vi "Save Extra data.vi"(2 "Temps":dbl[][](array[numeric]), 3 "Pixel Num.":i32, 4 "Save data Title":T1(ring), 5 "name or relative path":path) -> ()   [LabVIEW 2024]
uses:
  <vilib>/Utility/file.llb/Write Delimited Spreadsheet (string).vi
  <vilib>/Utility/file.llb/Write Delimited Spreadsheet (DBL).vi
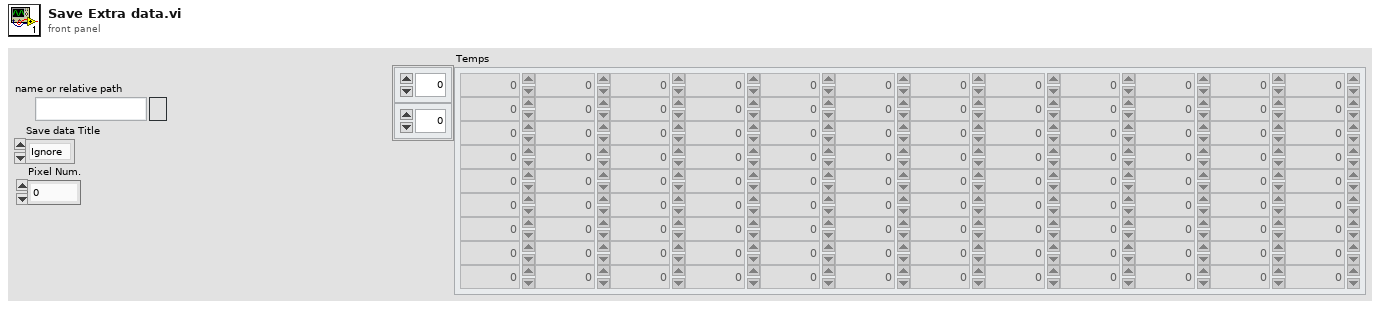
[diagram p1: front panel]
types:
  T1 = enum16{"Ignore", "All Wells Mean", "Pixel Values Wells"}
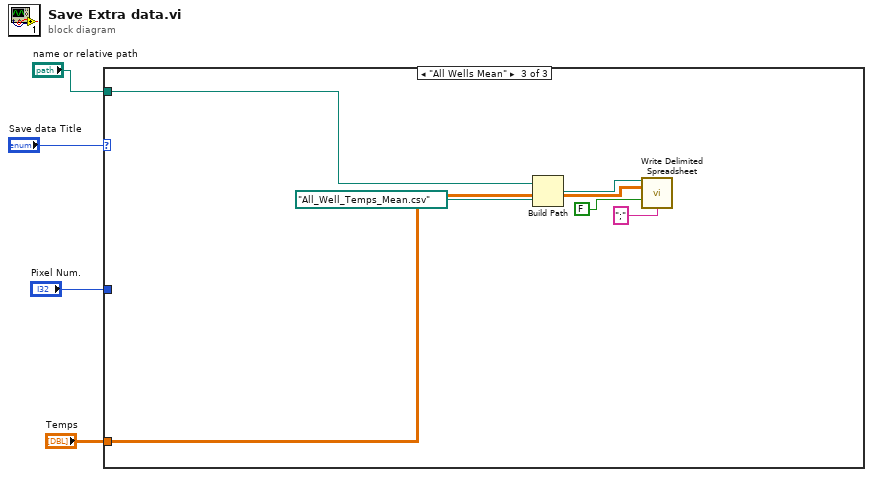
[diagram p0: block diagram]
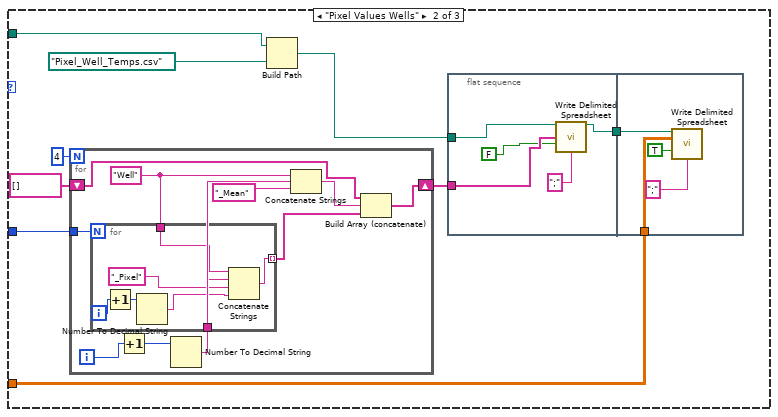
[diagram p3: hidden frame]
diagram:
  n1 = case shown="\"All Wells Mean\"" "Save data Title" {
    tunnel: "name or relative path" -> [_ w13 w43]
    tunnel: "Temps" -> [_ w9 w42]
    tunnel: "Pixel Num." -> [_ w8 _]
    frame "Ignore", Default {
    }
    frame "Pixel Values Wells" {
      n2 = for {
        N: 4 -> [_]
        tunnel: w8 -> [w23]
        shift-right: [w14] -> w6
        shift-left: string[] [] -> [w15]
        i -> [w21]
        w19 = "Well"
        n3 = Increment(x=w21) -> (x+1=w22:i32)
        n4 = Number To Decimal String(number=w22) -> (decimal integer string=w18:string)  [unwired: 1 in]
        n5 = for {
          N: w23 -> [_]
          tunnel: [w29] -> w16 mode=indexing
          tunnel: w19 -> [w27]
          tunnel: w18 -> [w26]
          i -> [w24]
          n6 = Increment(x=w24) -> (x+1=w25:i32)
          n7 = Number To Decimal String(number=w25) -> (decimal integer string=w28:string)  [unwired: 1 in]
          n8 = Concatenate Strings(w27, w26, "_Pixel", w28) -> (w29:string)
        }
        n9 = Concatenate Strings(w19, w18, "_Mean" ("string")) -> (w17:string)
        n10 = Build Array (concatenate)(w15, w17, w16) -> (w14:string[])
      }
      n11 = Build Path(base path=w13, name or relative path=path "Pixel_Well_Temps.csv") -> (appended path=w12:path)
      n12 = flat-sequence {
        tunnel: w12 -> [w32]
        tunnel: [w34] -> w10
        tunnel: w6 -> [w33]
        tunnel: w10 -> [w38]
        tunnel: w9 -> [w36]
        frame #0 {
          n13 = call-poly <vilib>:"Write Delimited Spreadsheet.vi"("file path (dialog if empty)"=w32, "1D data"=w33, "append to file? (new file:F)"=FALSE, "delimiter (\\t)"=";" ("delimiter (\\t)")) -> ("new file path (Not A Path if cancelled)"=w34:path)  [unwired: 10 in, 1 out]
        }
        frame #1 {
          n14 = call-poly <vilib>:"Write Delimited Spreadsheet.vi"("file path (dialog if empty)"=w38, "2D data"=w36, "append to file? (new file:F)"=TRUE, "delimiter (\\t)"=";" ("delimiter (\\t)")) -> ()  [unwired: 10 in, 2 out]
        }
      }
    }
    frame "All Wells Mean" {
      n15 = Build Path(base path=w43, name or relative path=path "All_Well_Temps_Mean.csv") -> (appended path=w41:path)
      n16 = call-poly <vilib>:"Write Delimited Spreadsheet.vi"("file path (dialog if empty)"=w41, "2D data"=w42, "append to file? (new file:F)"=FALSE, "delimiter (\\t)"=";" ("delimiter (\\t)")) -> ()  [unwired: 10 in, 2 out]
    }
  }
